vi "moveBoth.vi"(7 "Monochromator in":T1={"Type"=enum."Oriel", "Wavelength (nm)"=0.0, "Grating, gr/mm"=enum."2400", "Grating mode"=enum."IR", "Spectrum mode"={"Spectrum mode?"=FALSE, "Start wavelength (nm)"=0.0, "End wavelength (nm)"=0.0, "Wavelength step (nm)"=0.0, "Wavelength array"=[], "array index"=0}, "PTI"={"Delay before read (ms)"=0, "Mono 1"={"Timeout (ms)"=0, "Resource Name"="", "Baud Rate"=0, "Data Bits"=0, "Parity"=0, "Stop Bits"=0, "Flow Control"=0}, "Mono 2"={"Timeout (ms)"=0, "Resource Name"="", "Baud Rate"=0, "Data Bits"=0, "Parity"=0, "Stop Bits"=0, "Flow Control"=0}, "Two PTI Monochromators?"=FALSE}, "Oriel (custom)"={"reference"=refnum}, "Force wavelength confirmation (PTI)?"=FALSE} {"PTI"."Mono 2"."Flow Control" items=["1.0"=10, "1.5"=15, "2.0"=20]; "PTI"."Mono 2"."Stop Bits" items=["None", "Odd", "Even", "Mark", "Space"]; "PTI"."Mono 2"."Parity" items=["None", "Odd", "Even", "Mark", "Space"]; "PTI"."Mono 1"."Flow Control" items=["1.0"=10, "1.5"=15, "2.0"=20]; "PTI"."Mono 1"."Stop Bits" items=["None", "Odd", "Even", "Mark", "Space"]; "PTI"."Mono 1"."Parity" items=["None", "Odd", "Even", "Mark", "Space"]}, 8 "error in (no error)":errorcluster, 10 "Debug messages?":bool, 11 "wavelength":dbl) -> (0 "error out":errorcluster, 5 "Monochromator out":T1={"Type"=enum."Oriel", "Wavelength (nm)"=0.0, "Grating, gr/mm"=enum."2400", "Grating mode"=enum."IR", "Spectrum mode"={"Spectrum mode?"=FALSE, "Start wavelength (nm)"=0.0, "End wavelength (nm)"=0.0, "Wavelength step (nm)"=0.0, "Wavelength array"=[], "array index"=0}, "PTI"={"Delay before read (ms)"=0, "Mono 1"={"Timeout (ms)"=0, "Resource Name"="", "Baud Rate"=0, "Data Bits"=0, "Parity"=0, "Stop Bits"=0, "Flow Control"=0}, "Mono 2"={"Timeout (ms)"=0, "Resource Name"="", "Baud Rate"=0, "Data Bits"=0, "Parity"=0, "Stop Bits"=0, "Flow Control"=0}, "Two PTI Monochromators?"=FALSE}, "Oriel (custom)"={"reference"=refnum}, "Force wavelength confirmation (PTI)?"=FALSE} {"PTI"."Mono 2"."Flow Control" items=["1.0"=10, "1.5"=15, "2.0"=20]; "PTI"."Mono 2"."Stop Bits" items=["None", "Odd", "Even", "Mark", "Space"]; "PTI"."Mono 2"."Parity" items=["None", "Odd", "Even", "Mark", "Space"]; "PTI"."Mono 1"."Flow Control" items=["1.0"=10, "1.5"=15, "2.0"=20]; "PTI"."Mono 1"."Stop Bits" items=["None", "Odd", "Even", "Mark", "Space"]; "PTI"."Mono 1"."Parity" items=["None", "Odd", "Even", "Mark", "Space"]})   [LabVIEW 2017, in "Monochromator.lvlib" / "PTI.lvlib"]
uses:
  PTI.lvlib
  Controls/Params.ctl
  Controls/Type.ctl
  Controls/GratingValues.ctl
  Controls/Grating.ctl
  Controls/VISA parameters.ctl
  Custom Oriel drivers/Controls/Params.ctl
  C:/Optical Software Code V1.6.1.2/Optical Software Code/Modules/Monochromator/Cornerstone.dll
  Cornerstone.dll
  Monochromator.lvlib
  Serial comms/Serial comms.lvlib
  Custom Oriel drivers/Oriel (custom drivers).lvlib
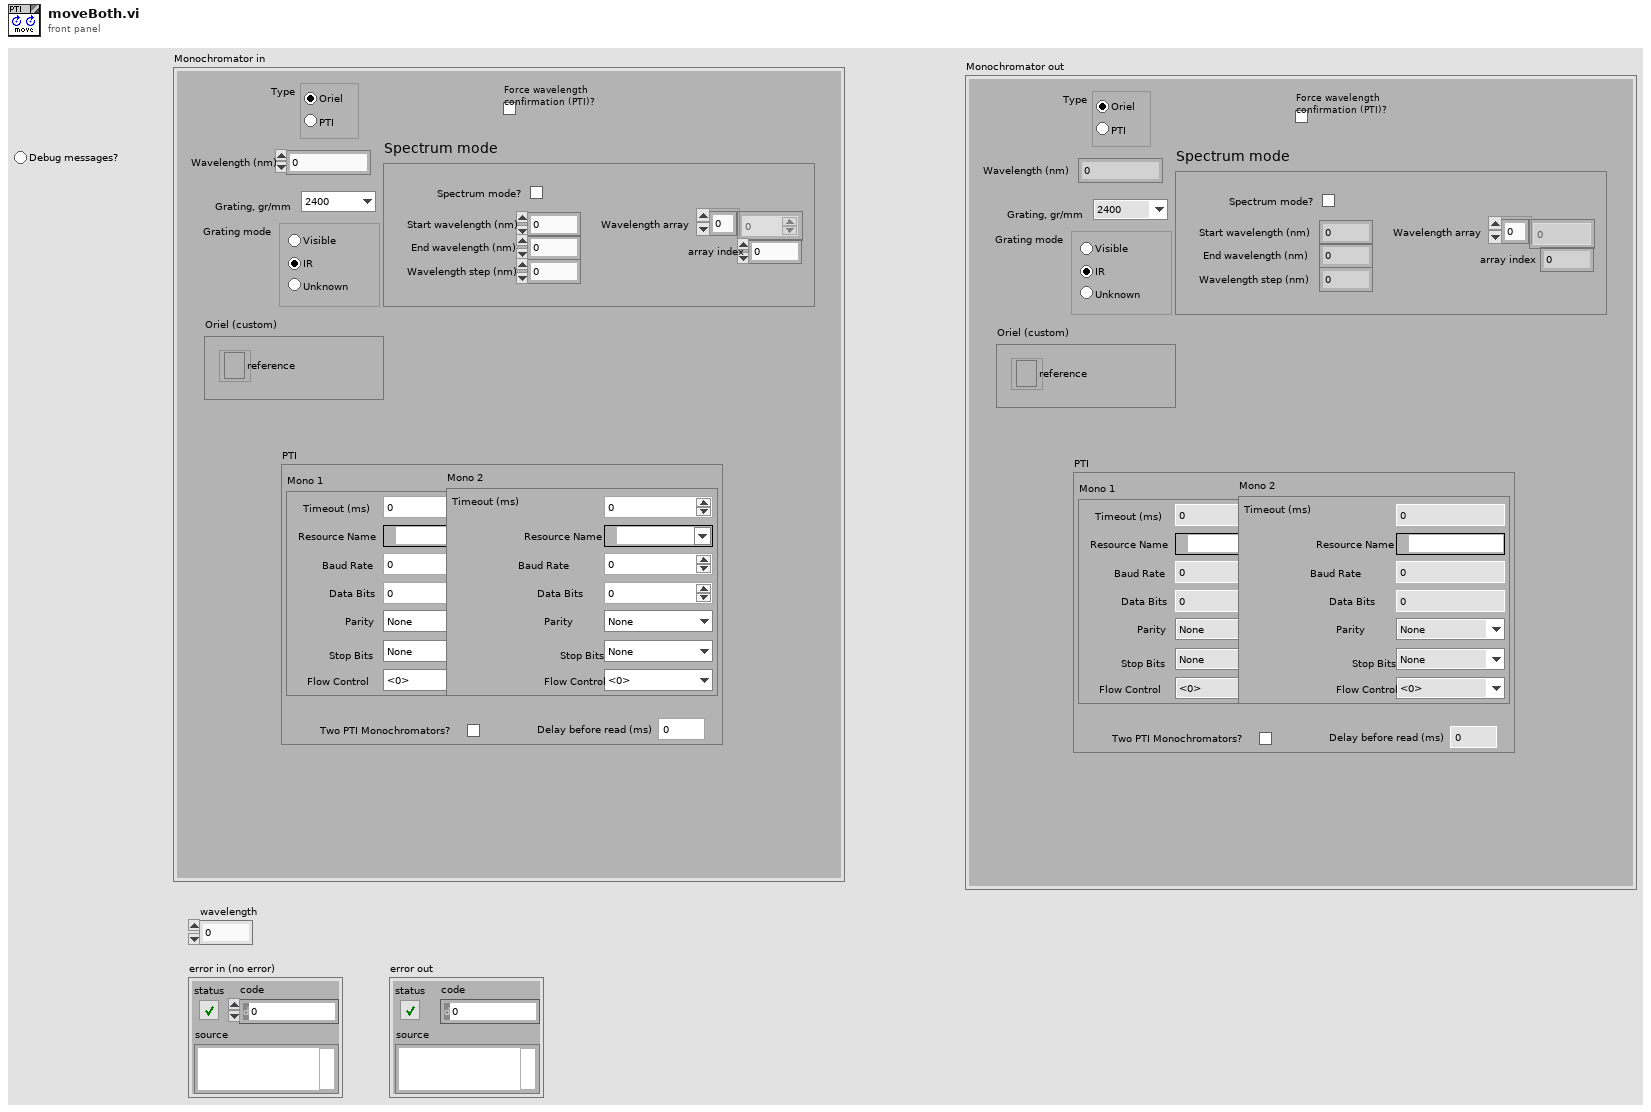
[diagram p1: front panel]
types:
  T1 = typedef "Monochromator.lvlib/Params.ctl" = cluster{"Type":T2, "Wavelength (nm)":dbl, "Grating, gr/mm":T3, "Grating mode":T4, "Spectrum mode":cluster{"Spectrum mode?":bool, "Start wavelength (nm)":dbl, "End wavelength (nm)":dbl, "Wavelength step (nm)":dbl, "Wavelength array":dbl[], "array index":u32}, "PTI":T5, "Oriel (custom)":T7, "Force wavelength confirmation (PTI)?":bool}
  T2 = typedef "Monochromator.lvlib/Type.ctl" = enum32{"Oriel", "PTI"}
  T3 = typedef "Monochromator.lvlib/GratingValues.ctl" = enum16{"2400", "1800", "1200", "600", "300", "150"}
  T4 = typedef "Monochromator.lvlib/Grating.ctl" = enum32{"Unknown", "Visible", "IR"}
  T5 = typedef "Monochromator.lvlib/PTI.lvlib/Params.ctl" = cluster{"Delay before read (ms)":u32, "Mono 1":T6, "Mono 2":T6, "Two PTI Monochromators?":bool}
  T6 = typedef "Serial comms.lvlib/VISA parameters.ctl" = cluster{"Timeout (ms)":u32, "Resource Name":refnum<visa-resource-name>, "Baud Rate":u32, "Data Bits":u16, "Parity":u16, "Stop Bits":u16, "Flow Control":u16}
  T7 = typedef "Monochromator.lvlib/Oriel (custom drivers).lvlib/Params.ctl" = cluster{"reference":refnum<k24>}
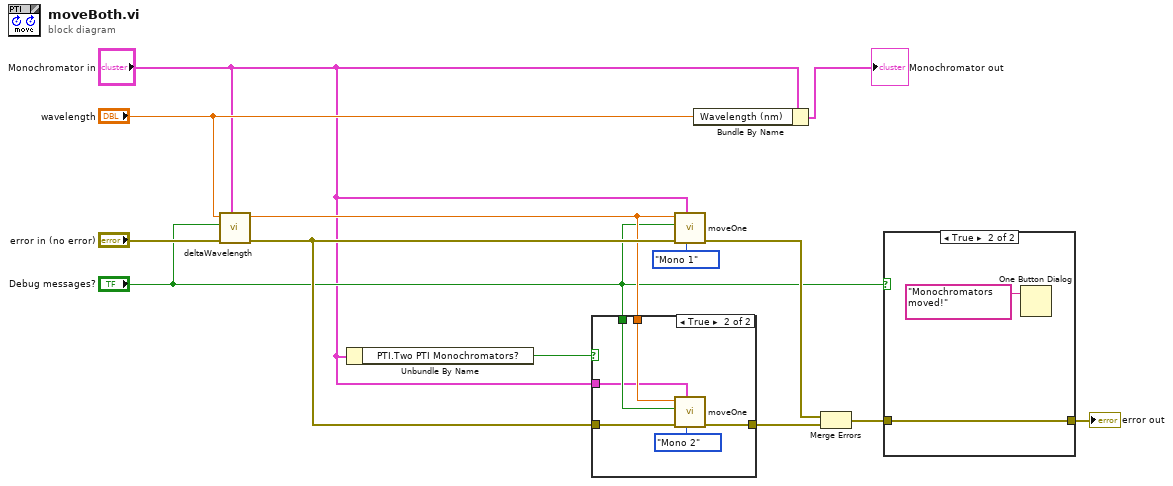
[diagram p0: block diagram]
diagram:
  n1 = call "deltaWavelength.vi"("Monochromator"="Monochromator in", "error in (no error)"="error in (no error)", "Debug messages?"="Debug messages?", "destination wavelength"="wavelength") -> ("error out"=w11:errorcluster, "delta wavelength"=w8:dbl)  [unwired: 6 in]
  n2 = Unbundle By Name("Monochromator in") -> ("PTI.Two PTI Monochromators?"=w1:bool)
  n3 = case shown="True" w1 {
    tunnel: w11 -> [w14 w20]
    tunnel: [w14 w19] -> w10
    tunnel: w8 -> [_ w18]
    tunnel: "Debug messages?" -> [_ w17]
    tunnel: "Monochromator in" -> [_ w15]
    frame False {
    }
    frame True {
      n4 = call "moveOne.vi"("Which mono"=enum16{"Mono 1", "Mono 2"}."Mono 2", "Monochromator"=w15, "error in (no error)"=w20, "Debug messages?"=w17, "Delta wavelength (nm)"=w18) -> ("error out"=w19:errorcluster)  [unwired: 6 in]
    }
  }
  n5 = call "moveOne.vi"("Which mono"=enum16{"Mono 1", "Mono 2"}."Mono 1", "Monochromator"="Monochromator in", "error in (no error)"=w11, "Debug messages?"="Debug messages?", "Delta wavelength (nm)"=w8) -> ("error out"=w9:errorcluster)  [unwired: 6 in]
  n6 = Bundle By Name(cluster="Monochromator in", "Wavelength (nm)"="wavelength") -> (→"Monochromator out":T1)
  n7 = Merge Errors(w9, w10) -> (w4:errorcluster)
  n8 = case shown="True" "Debug messages?" {
    tunnel: w4 -> [w21 w23]
    tunnel: [w21 w23] -> w3
    frame False {
    }
    frame True {
      n9 = One Button Dialog(message="Monochromators moved!") -> ()  [unwired: 1 in, 1 out]
    }
  }
  "error out" <- w3
